vi "Get Menus.vi"(8 "error in (no error)":errorcluster, 11 "Name":string) -> (0 "error out":errorcluster, 2 "Right Menu":T1, 3 "Left Menu":T1)   [LabVIEW 8.6]
doc: "This VI provides access to the defined set of menus, returning whichever is requested by the caller. It provides encapsulation of the menu list, so the list can be updated/modified without having to change this function or its callers."
uses:
  Controls/Menu.ctl
  Controls/Menus.ctl
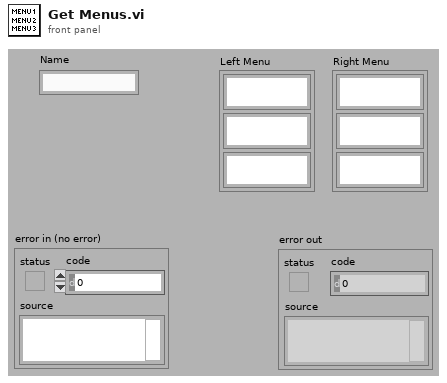
[diagram p1: front panel]
types:
  T1 = typedef "Menu.ctl" = cluster{"Menu 0":string, "Menu 1":string, "Menu 2":string}
  T2 = typedef "Menus.ctl" = cluster{"Menu Name":string, "Left Menu":T1, "Right Menu":T1}[]
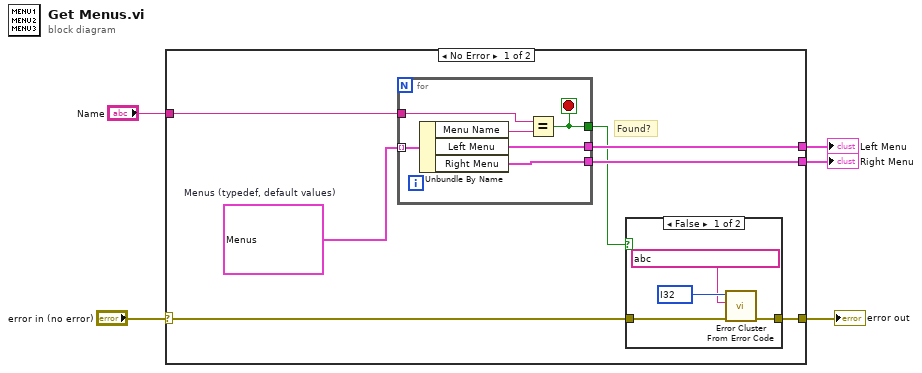
[diagram p0: block diagram]
diagram:
  n1 = case shown="No Error" "error in (no error)" {
    selector: "error in (no error)" -> [w6 w24]
    tunnel: "Name" -> [w12 _]
    tunnel: [w10 _] -> w4
    tunnel: [w9 _] -> w3
    tunnel: [w7 w24] -> w2
    frame #0 {
      w11 = T2 ?  # Menus (typedef, default values)
      # "Found?"
      n2 = for {
        tunnel: w11 -> [w23] mode=indexing
        tunnel: w12 -> [w21]
        tunnel: [w20] -> w8
        tunnel: [w19] -> w10
        tunnel: [w18] -> w9
        stop <- w20 stop-if-true
        n3 = Unbundle By Name(w23) -> ("Menu Name"=w22:string, "Left Menu"=w19:T1, "Right Menu"=w18:T1)
        n4 = Equal?(x=w21, y=w22) -> (x = y?=w20:bool)
      }
      n5 = case shown="False" w8 {
        tunnel: w6 -> [w16 w17]
        tunnel: [w15 w17] -> w7
        frame #0 {
          n6 = call <vilib>:"Error Cluster From Error Code.vi"("error in (no error)"=w16, "error message (\"\")"=string ? ("error message (\"\")"), "error code (0)"=i32 ?) -> ("error out"=w15:errorcluster)  [unwired: 6 in]
        }
        frame #1 {
        }
      }
    }
    frame #1 {
    }
  }
  "error out" <- w2
  "Left Menu" <- w4
  "Right Menu" <- w3
